vi "Testing.vi"(8 "error in (no error)":errorcluster, 11 "Cache Manager DVR in":refnum<class "Cache Manager.lvclass">) -> (0 "error out":errorcluster, 3 "Cache Manager DVR out":refnum<class "Cache Manager.lvclass">)   [LabVIEW 2020, in "Cache Manager.lvclass"]
uses:
  Cache Manager.lvclass
  Cache Manager.lvclass/Cache Manager.ctl
  Serializer/Serializable Message/Serializable Msg.lvclass
panel:
  out "Elapsed time (ms)":u32
  out "Array 2":string[](array[string])
  in  "Array":string[](array[string])=["Chat Window.lvlib:echo Msg.lvclass", "Chat Window.lvlib:echo Msg.lvclass", "Chat Window.lvlib:echo Reply Msg.lvclass", "Chat Window.lvlib:Display Text.lvclass"]
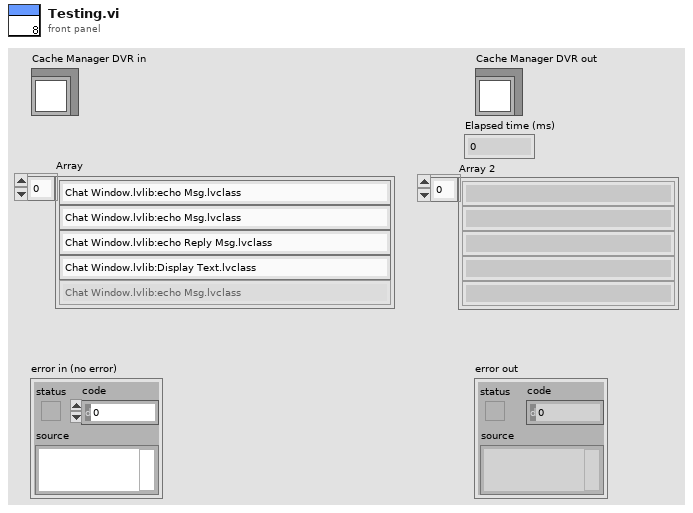
[diagram p1: front panel]
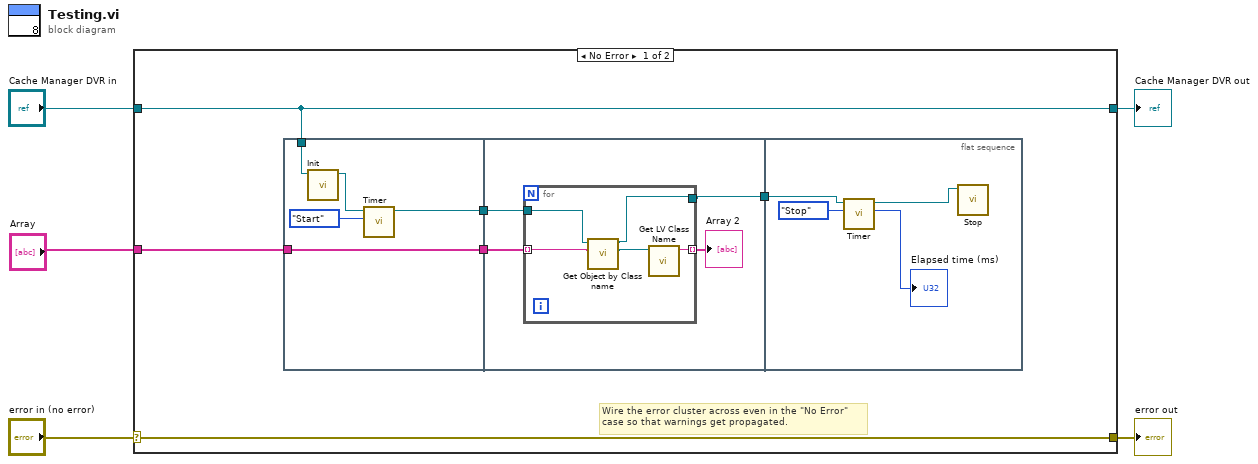
[diagram p0: block diagram]
diagram:
  n1 = case shown="No Error" "error in (no error)" {
    selector: "error in (no error)" -> [w11 w31]
    tunnel: [w11 w31] -> w4
    tunnel: [w8 w30] -> w2
    tunnel: "Cache Manager DVR in" -> [w8 w30]
    tunnel: "Array" -> [w10 _]
    frame No Error {
      # "Wire the error cluster across even in the \"No Error\"\ncase so that warnings get propagated."
      n2 = flat-sequence {
        tunnel: w10 -> [w16]
        tunnel: [w16] -> w9
        tunnel: w8 -> [w14]
        tunnel: [w12] -> w7
        tunnel: w9 -> [w20]
        tunnel: w7 -> [w18]
        tunnel: [w17] -> w6
        tunnel: w6 -> [w27]
        frame #0 {
          n3 = call "Init.vi"("Cache Manager DVR in"=w14) -> ("Cache Manager DVR out"=w13:refnum<class "Cache Manager.lvclass">)  [unwired: 9 in, 1 out]
          n4 = call "Timer.vi"("Action"=enum16{"Stop", "Start", ""}."Start", "Cache Manager DVR in"=w13) -> ("Cache Manager DVR out"=w12:refnum<class "Cache Manager.lvclass">)  [unwired: 7 in, 2 out]
        }
        frame #1 {
          n5 = for {
            tunnel: w20 -> [w23] mode=indexing
            tunnel: [w25] -> w19 mode=indexing
            tunnel: w18 -> [w24]
            tunnel: [w21] -> w17
            n6 = call "Get Object by Class name.vi"("Class name"=w23, "Cache Manager DVR in"=w24) -> ("Serialize out"=w22:refnum<class "Serializable Msg.lvclass">, "Cache Manager DVR out"=w21:refnum<class "Cache Manager.lvclass">)  [unwired: 7 in, 1 out]
            n7 = call <vilib>:"Get LV Class Name.vi"("object"=w22) -> ("class name"=w25:string)  [unwired: 9 in, 1 out]
          }
          "Array 2" <- w19
        }
        frame #2 {
          n8 = call "Timer.vi"("Action"=enum16{"Stop", "Start", ""}."Stop", "Cache Manager DVR in"=w27) -> ("Elapsed time (ms)"=→"Elapsed time (ms)":u32, "Cache Manager DVR out"=w26:refnum<class "Cache Manager.lvclass">)  [unwired: 7 in, 1 out]
          n9 = call "Stop.vi"("Cache Manager DVR in"=w26) -> ()  [unwired: 9 in, 2 out]
        }
      }
    }
    frame Error {
    }
  }
  "error out" <- w4
  "Cache Manager DVR out" <- w2
